vi "CheckLaserSTS.vi"() -> (0 "error out":errorcluster)   [LabVIEW 2019, in "MPC_Laser Marked.lvclass"]
uses:
  MPC_Laser Marked.lvclass
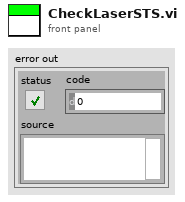
[diagram p1: front panel]
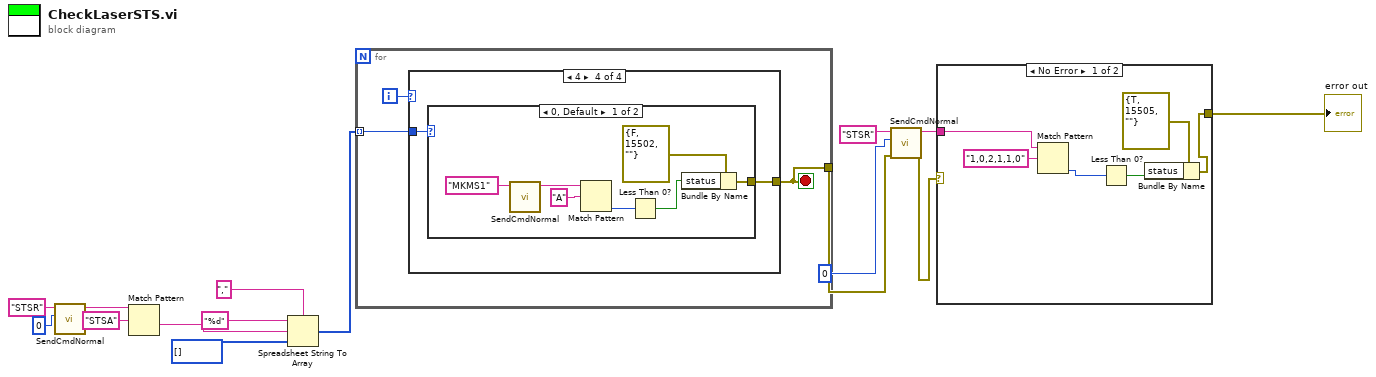
[diagram p0: block diagram]
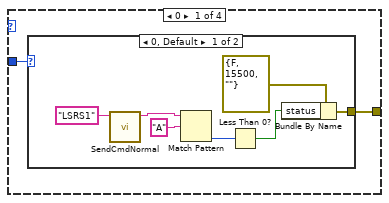
[diagram p3: hidden frame]
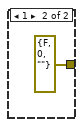
[diagram p4: hidden frame]
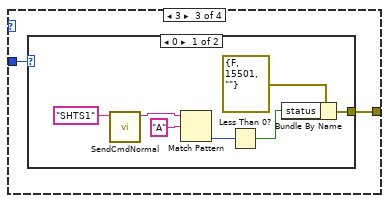
[diagram p7: hidden frame]
diagram:
  n1 = call "SendCmdNormal.vi"("index"=0, "DataIn"="STSR") -> ("Reccmd"=w3:string)  [unwired: 7 in, 2 out]
  n2 = Match Pattern(string=w3, regular expression="STSA") -> (after substring=w5:string)  [unwired: 1 in, 3 out]
  n3 = Spreadsheet String To Array(delimiter (Tab)=",", format string="%d", spreadsheet string=w5, array type (2D Dbl)=i32[] []) -> (array=w9:i32[])
  n4 = for {
    tunnel: w9 -> [w18] mode=indexing
    tunnel: [w16] -> w12
    i -> [w17]
    stop <- w16 stop-if-true
    n5 = case shown="4" w17 {
      tunnel: w18 -> [w20 w29 w31 w40]
      tunnel: [w19 _ w30 w39] -> w16
      frame 0 {
        n6 = case shown="0, Default" w20 {
          tunnel: [w22 errorcluster {"status"=FALSE, "code"=0, "source"=""} ("error out")] -> w19
          frame 0, Default {
            n7 = call "SendCmdNormal.vi"("DataIn"="LSRS1") -> ("Reccmd"=w26:string)  [unwired: 8 in, 2 out]
            n8 = Match Pattern(string=w26, regular expression="A") -> (offset past match=w24:i32)  [unwired: 1 in, 3 out]
            n9 = Less Than 0?(x=w24) -> (x < 0?=w21:bool)
            n10 = Bundle By Name(cluster=errorcluster {"status"=FALSE, "code"=15500, "source"=""} ("error constant"), "status"=w21) -> (w22:errorcluster)
          }
          frame 1 {
          }
        }
      }
      frame 1, Default {
        n11 = case shown="0, Default" w29 {
          frame 0, Default {
          }
          frame 1 {
          }
        }
      }
      frame 3 {
        n12 = case shown="0" w31 {
          tunnel: [w32 _] -> w30
          frame 0 {
            n13 = call "SendCmdNormal.vi"("DataIn"="SHTS1") -> ("Reccmd"=w38:string)  [unwired: 8 in, 2 out]
            n14 = Match Pattern(string=w38, regular expression="A") -> (offset past match=w37:i32)  [unwired: 1 in, 3 out]
            n15 = Less Than 0?(x=w37) -> (x < 0?=w36:bool)
            n16 = Bundle By Name(cluster=errorcluster {"status"=FALSE, "code"=15501, "source"=""} ("error constant"), "status"=w36) -> (w32:errorcluster)
          }
          frame 1, Default {
          }
        }
      }
      frame 4 {
        n17 = case shown="0, Default" w40 {
          tunnel: [w41 _] -> w39
          frame 0, Default {
            n18 = call "SendCmdNormal.vi"("DataIn"="MKMS1") -> ("Reccmd"=w47:string)  [unwired: 8 in, 2 out]
            n19 = Match Pattern(string=w47, regular expression="A") -> (offset past match=w46:i32)  [unwired: 1 in, 3 out]
            n20 = Less Than 0?(x=w46) -> (x < 0?=w45:bool)
            n21 = Bundle By Name(cluster=errorcluster {"status"=FALSE, "code"=15502, "source"=""} ("error constant"), "status"=w45) -> (w41:errorcluster)
          }
          frame 1 {
          }
        }
      }
    }
  }
  n22 = call "SendCmdNormal.vi"("error in (no error)"=w12, "index"=0, "DataIn"="STSR") -> ("error out"=w13:errorcluster, "Reccmd"=w14:string)  [unwired: 6 in, 1 out]
  n23 = case shown="No Error" w13 {
    selector: w13 -> [_ w54]
    tunnel: w14 -> [w53 _]
    tunnel: [w48 w54] -> w15
    frame No Error {
      n24 = Match Pattern(string=w53, regular expression="1,0,2,1,1,0") -> (offset past match=w51:i32)  [unwired: 1 in, 3 out]
      n25 = Less Than 0?(x=w51) -> (x < 0?=w50:bool)
      n26 = Bundle By Name(cluster=errorcluster {"status"=TRUE, "code"=15505, "source"=""} ("error constant"), "status"=w50) -> (w48:errorcluster)
    }
    frame Error {
    }
  }
  "error out" <- w15
